vi "Open CANCoders.vi"(8 "error in":errorcluster, 11 "CANCoder Can IDs":T3={"LF ID"=12, "LB ID"=11, "RF ID"=10, "RB ID"=9}) -> (0 "error out":errorcluster)   [LabVIEW 2020]
uses:
  ctl/Swerve Absolute Encoders.ctl
  ctl/Absolute Encoder Type.ctl
panel:
  out "Swerve CANCoders":T1
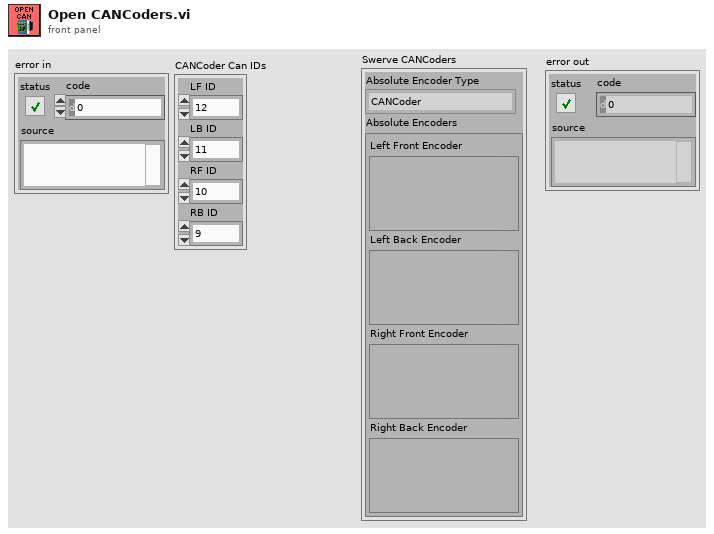
[diagram p1: front panel]
types:
  T1 = typedef "Swerve Absolute Encoders.ctl" = cluster{"Absolute Encoder Type":T2, "Absolute Encoders":cluster{"Left Front Encoder":variant, "Left Back Encoder":variant, "Right Front Encoder":variant, "Right Back Encoder":variant}}
  T2 = typedef "Absolute Encoder Type.ctl" = enum16{"CANCoder", "Through Bore Encoder"}
  T3 = cluster{"LF ID":u8, "LB ID":u8, "RF ID":u8, "RB ID":u8}
  T4 = typedef "CTRE_Phoenix_CANcoder_DeviceRef.ctl" = cluster{"DeviceStatus":errorcluster, "Device Number":u8, "Handle":u64, "UsageFrame":u32, "Library Path":path}
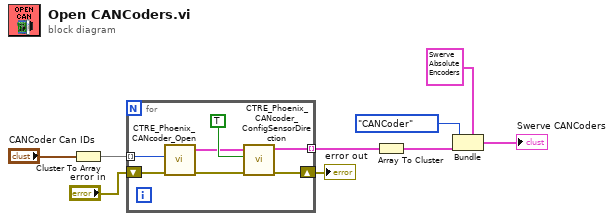
[diagram p0: block diagram]
diagram:
  n1 = Cluster To Array(cluster="CANCoder Can IDs") -> (array=w8:u8[])
  n2 = for {
    tunnel: w8 -> [w16] mode=indexing
    shift-right: [w11] -> w6
    shift-left: "error in" -> [w15]
    tunnel: [w12] -> w4 mode=indexing
    n3 = call <vilib>:"CTRE_Phoenix_CANcoder_Open.vi"("error in"=w15, "Device Number"=w16) -> ("error out"=w10:errorcluster, "CTRE_CANcoder_DeviceRef"=w13:T4)  [unwired: 8 in]
    n4 = call <vilib>:"CTRE_Phoenix_CANcoder_ConfigSensorDirection.vi"("error in"=w10, "Sensor Direction"=TRUE, "CTRE_CANcoder_DeviceRef"=w13) -> ("error out"=w11:errorcluster, "CTRE_CANcoder_DeviceRef"=w12:T4)  [unwired: 7 in]
  }
  "error out" <- w6
  n5 = Array To Cluster(array=w4) -> (cluster=w3:cluster{"[0]":T4, "[1]":T4, "[2]":T4, "[3]":T4})
  n6 = Bundle(cluster=T1 {"Absolute Encoder Type"=enum."CANCoder", "Absolute Encoders"={"Left Front Encoder"=variant, "Left Back Encoder"=variant, "Right Front Encoder"=variant, "Right Back Encoder"=variant}} ("Absolute Encoders"), "Absolute Encoder Type"=Absolute_Encoder_Type."CANCoder", "Absolute Encoders"=w3) -> (→"Swerve CANCoders":T1)
